vi "led_lcd.vi"() -> ()   [LabVIEW 2016]
panel:
  in  "VISA resource name":refnum<visa-resource-name>
  out "error out":errorcluster
  in  "stop":bool
  in  "write buffer":string
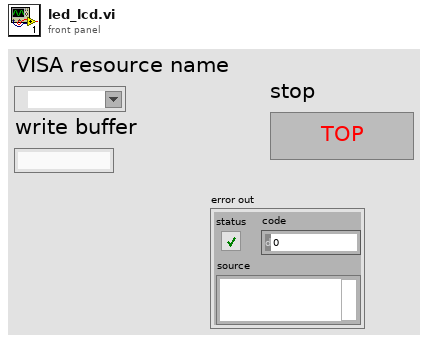
[diagram p1: front panel]
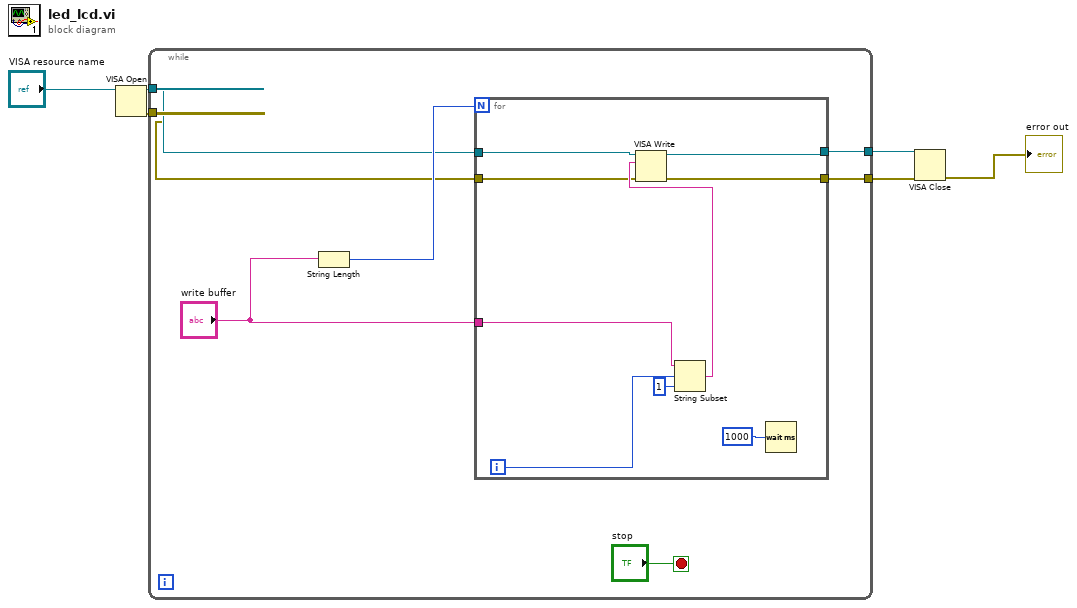
[diagram p0: block diagram]
diagram:
  n1 = VISA Open(VISA resource name="VISA resource name") -> (VISA resource name=w4:refnum<visa-resource-name>, error out=w3:errorcluster)  [unwired: 4 in]
  n2 = while {
    tunnel: w4 -> [w10]
    tunnel: w3 -> [w8]
    tunnel: [w9] -> w2
    tunnel: [w7] -> w1
    stop <- "stop" stop-if-true
    n3 = String Length(string="write buffer") -> (length=w12:i32)
    n4 = for {
      N: w12 -> [_]
      tunnel: "write buffer" -> [w21]
      tunnel: w10 -> [w19]
      tunnel: [w18] -> w9
      tunnel: w8 -> [w16]
      tunnel: [w15] -> w7
      i -> [w22]
      n5 = String Subset(string=w21, offset (0)=w22, length (rest)=1 ("length (rest)")) -> (substring=w17:string)
      n6 = VISA Write(VISA resource name=w19, write buffer=w17, error in (no error)=w16) -> (VISA resource name out=w18:refnum<visa-resource-name>, error out=w15:errorcluster)  [unwired: 1 out]
      n7 = Wait (ms)(milliseconds to wait=u32 1000 ("millisecond timer value")) -> ()  [unwired: 1 out]
    }
  }
  n8 = VISA Close(VISA resource name=w2, error in (no error)=w1) -> (error out=→"error out":errorcluster)
